vi "MasterAcquisitionFile_IOS_test.vi"() -> ()   [LabVIEW 2020]
uses:
  <vilib>/vision/driver/IMAQdx.llb/IMAQdx Acquisition Mode.ctl
  <vilib>/vision/driver/IMAQdx.llb/IMAQdx Camera Control Mode.ctl
  <vilib>/userDefined/High Color/IMAQdx.ctl
  <vilib>/vision/driver/IMAQdx.llb/IMAQdx Buffer Number Mode.ctl
  <vilib>/DAQmx/read.llb/DAQmx Read (Analog 1D Wfm NChan NSamp).vi
  <vilib>/Waveform/DWDTOps.llb/DWDT Digital to Boolean Array.vi
  <vilib>/DAQmx/create/channels.llb/DAQmx Create Channel (CO-Pulse Generation-Frequency).vi
  <vilib>/DAQmx/configure/timing.llb/DAQmx Timing (Implicit).vi
  <vilib>/DAQmx/create/channels.llb/DAQmx Create Channel (AI-Voltage-Basic).vi
  <vilib>/DAQmx/configure/timing.llb/DAQmx Timing (Sample Clock).vi
  <vilib>/DAQmx/configure/trigger.llb/DAQmx Start Trigger (Digital Edge).vi
  <vilib>/DAQmx/miscellaneous.llb/DAQmx Fill In Error Info.vi
  <vilib>/vision/driver/NI_Vision_Acquisition_Software.lvlib
  <resource>/objmgr/imaqdx.rc
panel:
  out "Saving":bool=TRUE
  in  "stop":bool
  in  "Sol Stim Parameters":cluster{"Fs":dbl, "Samples":dbl}
  in  "LED Stim Parameters":cluster{"Fs":dbl, "Samples":dbl}
  in  "Sol Duty Cycle (%)":dbl=10.0
  in  "Sol Freq":dbl=1.0
  in  "Sol Dur (s)":dbl=1.0
  in  "LED Duty Cycle (%)":dbl=10.0
  in  "LED Freq":dbl=10.0
  in  "LED Dur (s)":dbl=2.0
  out "Stimulus Order":digitalwaveform[](graph)=[{"t0"=timestamp(0 s since 1904-01-01), "dt"=5e-05, "Y"={"transitions"=[], "data"=array18001000x1[18001000 elements]}}, {"t0"=timestamp(0 s since 1904-01-01), "dt"=5e-05, "Y"={"transitions"=[], "data"=array18001000x1[18001000 elements]}}, {"t0"=timestamp(0 s since 1904-01-01), "dt"=5e-05, "Y"={"transitions"=[], "data"=array18001000x1[18001000 elements]}}, {"t0"=timestamp(0 s since 1904-01-01), "dt"=5e-05, "Y"={"transitions"=[], "data"=array18001000x1[18001000 elements]}}]
  out "Solenoid Stim":digitalwaveform(graph)={"t0"=timestamp(0 s since 1904-01-01), "dt"=5e-05, "Y"={"transitions"=[], "data"=array20000x1[20000 elements]}}
  in  "Trial Offset (s)":dbl=15.0
  in  "Interstim (s)":dbl=30.0
  in  "Right Pad":dbl=1.0
  in  "Left Pad":dbl=1.0
  in  "Auditory":dbl=1.0
  in  "LED":dbl
  out "?":T1(plugin-control)
  out "?":T1(plugin-control)
  out "Whisk Cam":bool=TRUE
  out "Web Cam":bool=TRUE
  out "Analog":bool=TRUE
  out "Web Cam Fs":dbl(knob)=29.86263189329086 scale=0.0..200.0
  out "Whisk Cam Fs":dbl(knob)=150.0 scale=0.0..200.0
  out "Dev1 Samples":i32=336839
  in  "Dev1 Analog Channels":string[](array[string])=["Cortical_LH", "Force_Sensor", "LPadSol", "RPadSol", "AudSol", "Hippocampus", "EMG", "Cortical_RH", "OptoLED"]
  in  "Analog Acquisition":cluster{"Analog Fs":u16}={"Analog Fs"=20000} {"Analog Fs" format="%0.0f"}
  in  "Sampling Rates":T2={"CBV Cam Fs"=30, "Whisk Cam Fs"=150, "Web Cam Fs"=30, "Pupil Cam Fs"=30}
  out "Notes Size":i32=8
  out "Notes Reversed":string[](array[string])=["Experimenter", "Animal ID", "Hemisphere", "Solenoid PSI", "Isoflurane time", "Session ID", "Amplifier Gain", "LED power (mW)"]
  out "Notes Array":string[](array[string])=["LED power (mW)", "Amplifier Gain", "Session ID", "Isoflurane time", "Solenoid PSI", "Hemisphere", "Animal ID", "Experimenter"]
  in  "Notes:":T3={"Experimenter"="Kevin", "Animal ID"="T195", "Hemisphere"="Both", "Solenoid PSI"="10", "Isoflurane time"="1130", "Session ID"="Imaging Session Five", "Amplifier Gain"="10000", "LED power (mW)"="10"}
  in  "Target Path":path=path "D:/T195/Imaging Session 5 - 5 June 2021" caption="Final Save Location"
  out "Dropped":u32(slide) caption="Whisk Cam" scale=0.0..999.0
  out "Filename":string="210605_11_36_30"
  in  "Time (min)":dbl(knob)=15.0 min=0.5 max=20.0 step=0.5 scale=0.0..20.0 scale format="%#_2g"
  in  "Temp Path":path=path "D:/LabVIEW Streamed Data" caption="Temporary Path for Streamed Data"
  out "Last Whisk\nBuffer":u32=2524
  # "Dropped Frames"
  # "Stimuli"
  # "LPAD"
  # "RPAD"
  # "AUD"
  # "LED"
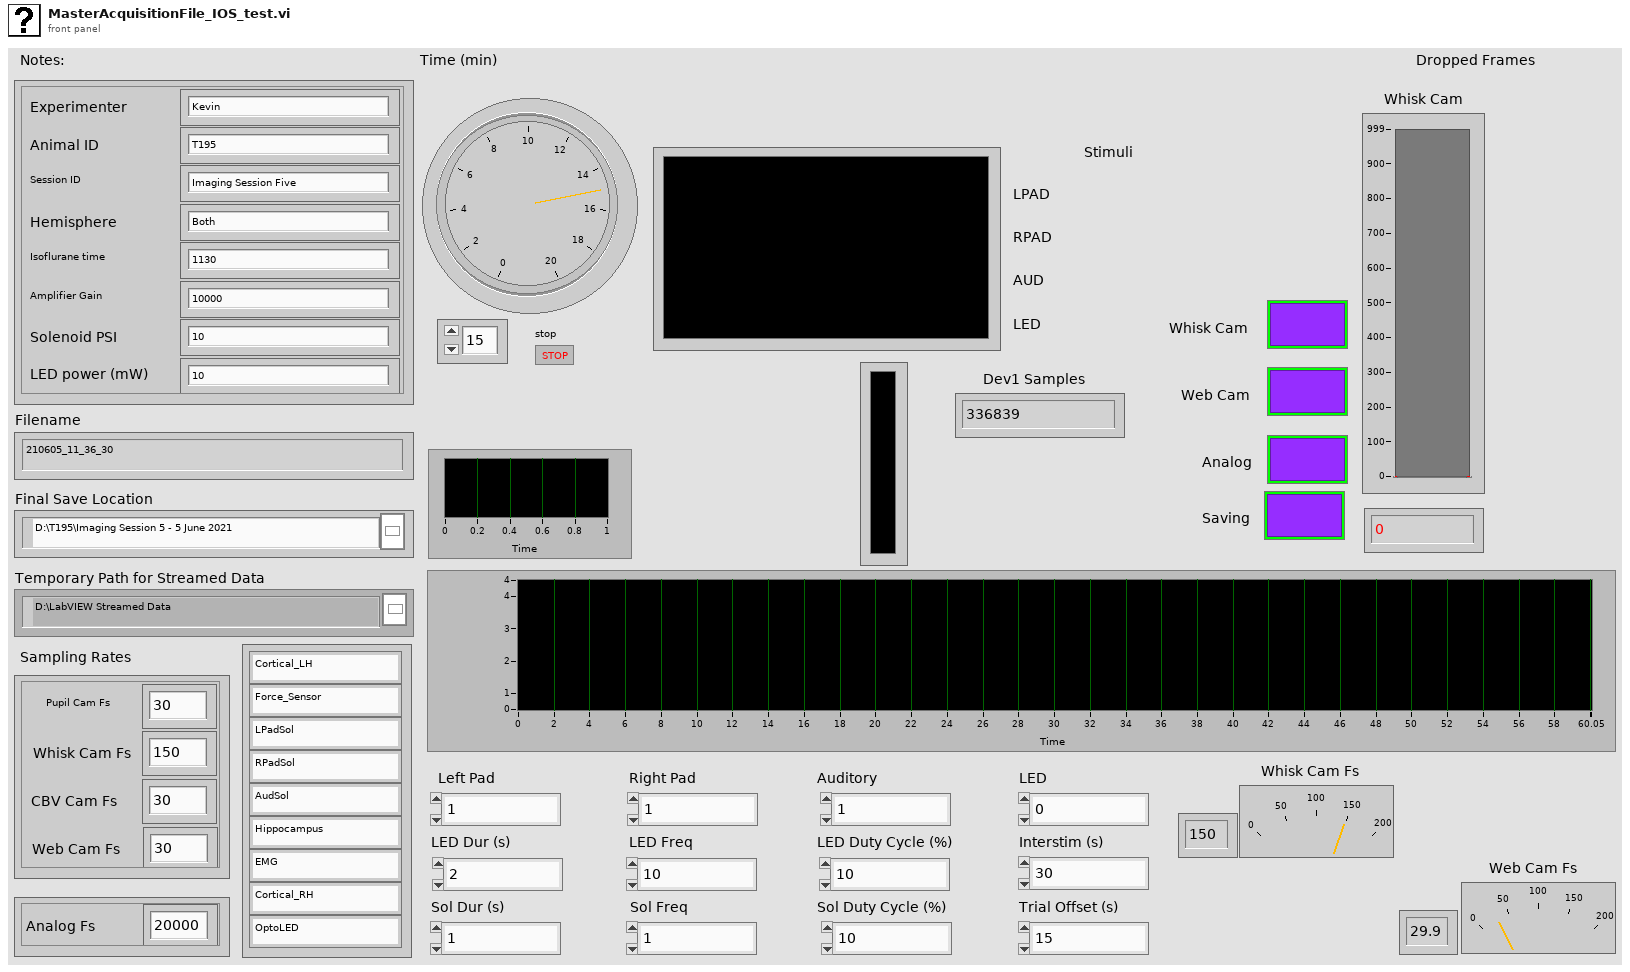
[diagram p1: front panel]
types:
  T1 = typedef "IMAQ Image.ctl" = refnum<image>
  T2 = cluster{"CBV Cam Fs":u16, "Whisk Cam Fs":u16, "Web Cam Fs":u16, "Pupil Cam Fs":u16}
  T3 = cluster{"Experimenter":string, "Animal ID":string, "Hemisphere":string, "Solenoid PSI":string, "Isoflurane time":string, "Session ID":string, "Amplifier Gain":string, "LED power (mW)":string}
  T4 = typedef "IMAQdx.ctl" = refnum<k21>
  T5 = enum16{"open", "open or create", "create or replace", "create", "open (read-only)"}
  T6 = typedef "Image Type" = u32
  T7 = typedef "NI_Vision_Acquisition_Software.lvlib/IMAQdx Camera Control Mode.ctl" = enum32{"Controller", "Listener"}
  T8 = enum16{"open", "replace", "create", "open or create", "replace or create", "replace or create with confirmation"}
  T9 = typedef "NI_Vision_Acquisition_Software.lvlib/IMAQdx Acquisition Mode.ctl" = enum32{"One Shot", "Continuous"}
  T10 = typedef "IMAQ AVI2 Refnum.ctl" = refnum<k20>
  T11 = enum16{"big-endian, network order", "native, host order", "little-endian"}
  T12 = typedef "NI_Vision_Acquisition_Software.lvlib/IMAQdx Buffer Number Mode.ctl" = enum32{"Next", "Last", "Buffer Number", "Every", "Last New"}
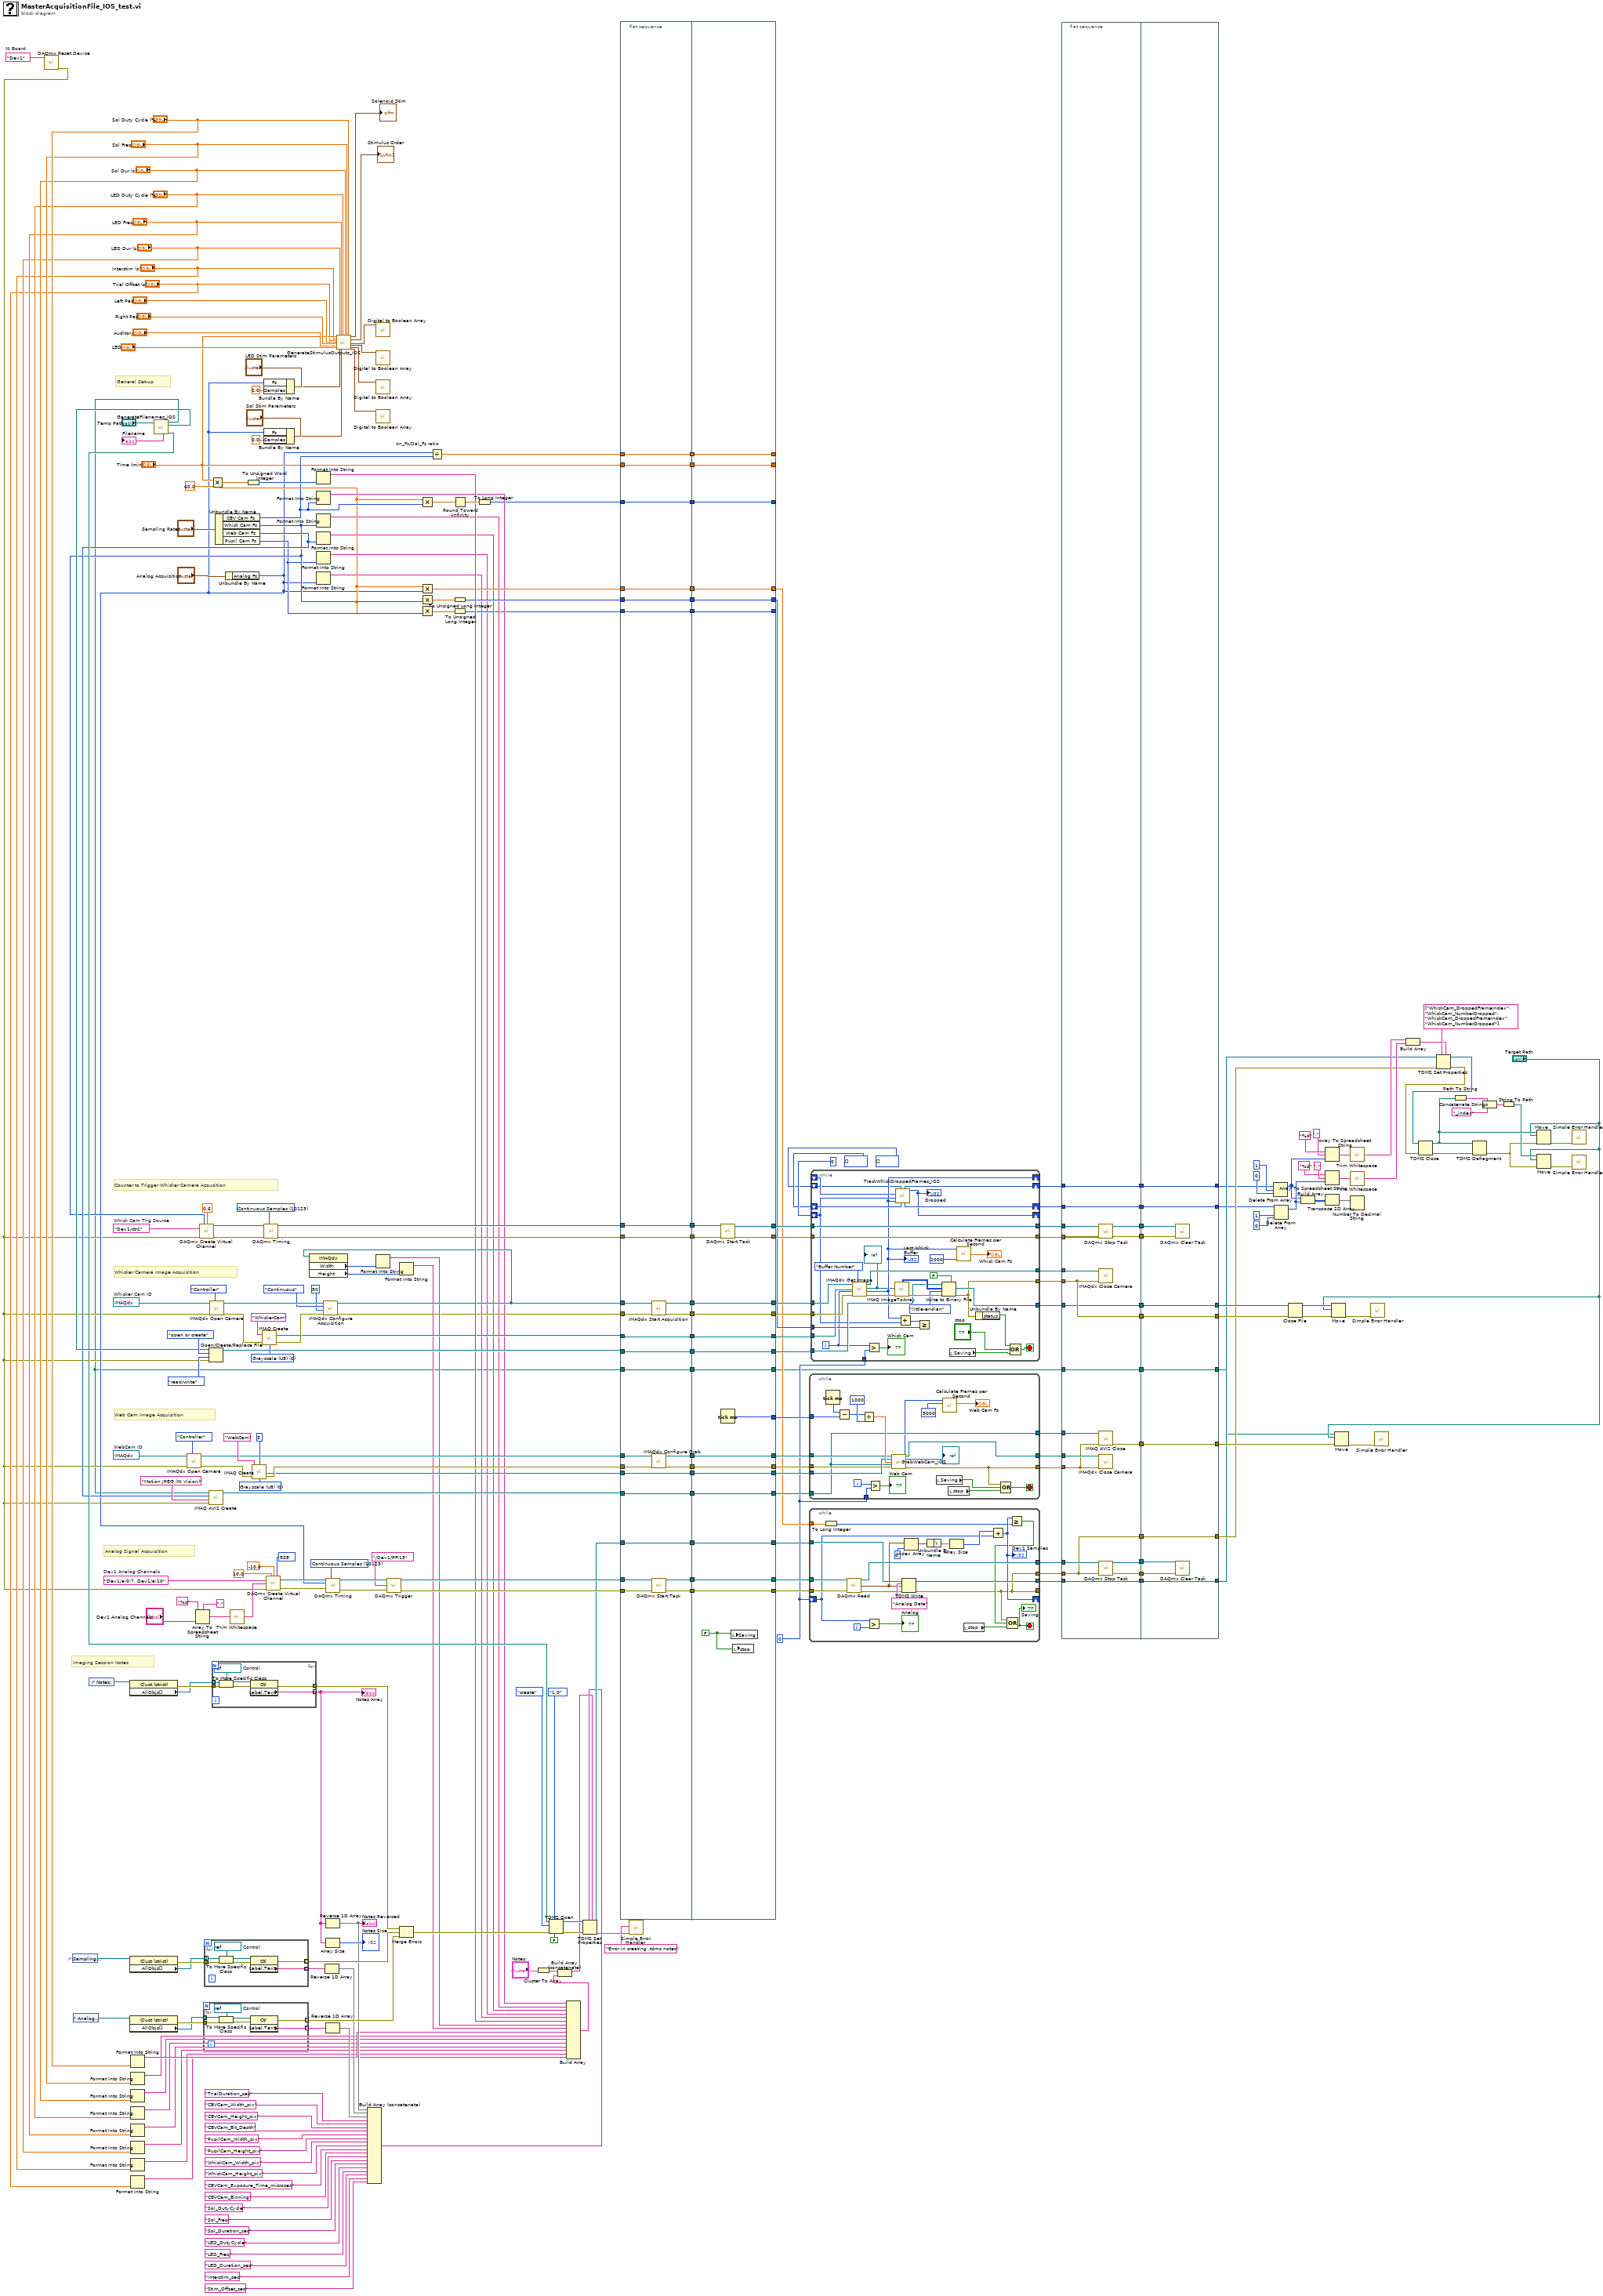
[diagram p0: block diagram]
diagram:
  w155 = tag "Dev1/ai0:7, Dev1/ai10"  # Dev1 Analog Channels
  w158 = T4 "cam0"  # WebCam ID
  w141 = T4 "cam1"  # Whisker Cam ID
  w268 = tag "Dev1/ctr1"  # Whisk Cam Trig Source
  w84 = 0
  w223 = 10123 items=["Finite Samples"=10178, "Continuous Samples"=10123, "Hardware Timed Single Point"=12522] ("sample mode")
  w226 = 10083 items=["default"=-1, "RSE"=10083, "NRSE"=10078, "Differential"=10106, "Pseudodifferential"=12529] ("input terminal configuration")
  w256 = T6 0 items=["Grayscale (U8)", "Grayscale (I16)", "Grayscale (SGL)", "Complex (CSG)", "RGB (U32)", "HSL (U32)", "RGB (U64)", "Grayscale (U16)"] ("Image Type")
  w263 = tag "Dev1"  # NI Board
  w264 = 10123 items=["Finite Samples"=10178, "Continuous Samples"=10123, "Hardware Timed Single Point"=12522] ("sample mode")
  w271 = T6 0 items=["Grayscale (U8)", "Grayscale (I16)", "Grayscale (SGL)", "Complex (CSG)", "RGB (U32)", "HSL (U32)", "RGB (U64)", "Grayscale (U16)"] ("Image Type")
  # "General Set-up"
  # "Whisker Camera Image Acquisition"
  # "Imaging Session Notes"
  # "Counter to Trigger Whisker Camera Acqusition"
  # "Web Cam Image Acquisition"
  # "Analog Signal Acquisition"
  n1 = call <vilib>:"DAQmx Reset Device.vi"("device in"=w263) -> ("error out"=w37:errorcluster)  [unwired: 14 in]
  n2 = control-ref of="Sampling Rates"() -> (w164:refnum<vi>)
  n3 = control-ref of="Analog Acquisition"() -> (w163:refnum<vi>)
  n4 = control-ref of="Notes:"() -> (w185:refnum<vi>)
  n5 = property class="Clust (strict)"(reference=w185) -> (error out=w188:errorcluster, "AllObjs[]"=w120:refnum<vi>[])  [unwired: 1 in, 1 out]
  n6 = property class="Clust (strict)"(reference=w164) -> (error out=w183:errorcluster, "AllObjs[]"=w121:refnum<vi>[])  [unwired: 1 in, 1 out]
  n7 = property class="Clust (strict)"(reference=w163) -> (error out=w162:errorcluster, "AllObjs[]"=w119:refnum<vi>[])  [unwired: 1 in, 1 out]
  n8 = Format Into String("Sol Duty Cycle (%)") -> (resulting string=w61:string)  [unwired: 3 in, 1 out]
  n9 = Format Into String("Sol Freq") -> (resulting string=w60:string)  [unwired: 3 in, 1 out]
  n10 = Format Into String("Sol Dur (s)") -> (resulting string=w59:string)  [unwired: 3 in, 1 out]
  n11 = Format Into String("LED Duty Cycle (%)") -> (resulting string=w58:string)  [unwired: 3 in, 1 out]
  n12 = Format Into String("LED Freq") -> (resulting string=w57:string)  [unwired: 3 in, 1 out]
  n13 = Format Into String("LED Dur (s)") -> (resulting string=w56:string)  [unwired: 3 in, 1 out]
  n14 = Format Into String("Interstim (s)") -> (resulting string=w55:string)  [unwired: 3 in, 1 out]
  n15 = Format Into String("Trial Offset (s)") -> (resulting string=w54:string)  [unwired: 3 in, 1 out]
  n16 = call "GenerateFilenames_IOS.vi"("path"="Temp Path") -> ("TDMS Path"=w180:path, "Basler Path"=w259:path, "WebCam Path"=w1:path, "Analog file name"=→"Filename":string)  [unwired: 3 in, 4 out]
  n17 = call <vilib>:"IMAQdx Open Camera.vi"("Camera Control Mode"=IMAQdx_Camera_Control_Mode."Controller", "error in"=w37, "Session In"=w158) -> ("error out"=w252:errorcluster, "Session Out"=w250:T4)  [unwired: 7 in]
  n18 = Array To Spreadsheet String(delimiter (Tab)=",", array="Dev1 Analog Channels", 3:"%s" ("format string")) -> (spreadsheet string=w152:string)
  n19 = for {
    tunnel: [w283] -> w160 mode=indexing
    tunnel: w162 -> [w282]
    tunnel: [w280] -> w161 mode=indexing
    tunnel: w119 -> [w279] mode=indexing
    w284 = refnum<vi> refnum  # Control
    n20 = To More Specific Class(target class=w284, reference=w279, error in=w282) -> (specific class reference=w285:refnum<vi>, error out=w281:errorcluster)
    n21 = property class="Ctl"(reference=w285, error in=w281) -> (error out=w280:errorcluster, "Label.Text"=w283:string)  [unwired: 1 out]
  }
  n22 = for {
    tunnel: [w290] -> w184 mode=indexing
    tunnel: w183 -> [w289]
    tunnel: [w287] -> w170 mode=indexing
    tunnel: w121 -> [w286] mode=indexing
    w291 = refnum<vi> refnum  # Control
    n23 = To More Specific Class(target class=w291, reference=w286, error in=w289) -> (specific class reference=w292:refnum<vi>, error out=w288:errorcluster)
    n24 = property class="Ctl"(reference=w292, error in=w288) -> (error out=w287:errorcluster, "Label.Text"=w290:string)  [unwired: 1 out]
  }
  n25 = Open/Create/Replace File(file path (use dialog)=w259, error in=w37, operation (0:open)=T8."open or create", access (0:read/write)=enum16{"read/write", "read-only", "write-only"}."read/write") -> (refnum out=w229:refnum<file>)  [unwired: 2 in, 2 out]
  n26 = call <vilib>:"IMAQdx Open Camera.vi"("Camera Control Mode"=IMAQdx_Camera_Control_Mode."Controller", "error in"=w37, "Session In"=w141) -> ("error out"=w274:errorcluster, "Session Out"=w277:T4)  [unwired: 7 in]
  n27 = Multiply(x="Time (min)", y=60.0) -> (x*y=w71:dbl)
  n28 = for {
    tunnel: [w297] -> w187 mode=indexing
    tunnel: w188 -> [w296]
    tunnel: [w294] -> w171 mode=indexing
    tunnel: w120 -> [w293] mode=indexing
    w298 = refnum<vi> refnum  # Control
    n29 = To More Specific Class(target class=w298, reference=w293, error in=w296) -> (specific class reference=w299:refnum<vi>, error out=w295:errorcluster)
    n30 = property class="Ctl"(reference=w299, error in=w295) -> (error out=w294:errorcluster, "Label.Text"=w297:string)  [unwired: 1 out]
  }
  "Notes Array" <- w187
  n31 = Unbundle By Name("Sampling Rates") -> ("CBV Cam Fs"=w72:u16, "Whisk Cam Fs"=w106:u16, "Web Cam Fs"=w157:u16, "Pupil Cam Fs"=w100:u16)
  n32 = call-poly <vilib>:"DAQmx Create Virtual Channel.vi"("frequency"=w106, "duty cycle"=0.6, "counter"=w268, "error in"=w37) -> ("task out"=w266:refnum<k21>, "error out"=w265:errorcluster)  [unwired: 10 in]
  n33 = call "IMAQ AVI2 Create"("error in (no error)"=w37, "Codec"="Motion JPEG (NI Vision)", "Frames Per Second"=w157, "AVI Path"=w1) -> ("AVI Refnum"=w242:T10)  [unwired: 6 in, 1 out]
  n34 = Unbundle By Name("Analog Acquisition") -> ("Analog Fs"=w45:u16)
  n35 = call <vilib>:"Trim Whitespace.vi"("string"=w152) -> ("trimmed string"=w151:string)  [unwired: 1 in]
  n36 = To Unsigned Word Integer(number=w71) -> (unsigned 16bit integer=w147:u16)
  n37 = call "IMAQ Create"("Border Size"=3, "Image Name"="WebCam", "Image Type"=w256, "error in (no error)"=w252) -> ("New Image"=w249:T1, "error out"=w251:errorcluster)  [unwired: 1 in]
  n38 = call "IMAQ Create"("Image Name"="WhiskerCam", "Image Type"=w271, "error in (no error)"=w274) -> ("New Image"=w139:T1, "error out"=w272:errorcluster)  [unwired: 2 in]
  n39 = Bundle By Name(cluster="LED Stim Parameters", "Fs"=w45, "Samples"=0.0) -> (w77:cluster{"Fs":dbl, "Samples":dbl})
  n40 = Bundle By Name(cluster="Sol Stim Parameters", "Fs"=w45, "Samples"=0.0) -> (w78:cluster{"Fs":dbl, "Samples":dbl})
  n41 = call-poly <vilib>:"DAQmx Timing.vi"("task/channels in"=w266, "sample mode"=w264, "error in"=w265) -> ("task out"=w213:refnum<k21>, "error out"=w211:errorcluster)  [unwired: 11 in]
  n42 = call-poly <vilib>:"DAQmx Create Virtual Channel.vi"("maximum value"=10.0, "minimum value"=-10.0, "input terminal configuration"=w226, "physical channels"=w155, "name to assign"=w151, "error in"=w37) -> ("task out"=w225:refnum<k21>, "error out"=w224:errorcluster)  [unwired: 8 in]
  n43 = Format Into String(w147) -> (resulting string=w149:string)  [unwired: 3 in, 1 out]
  n44 = Format Into String(w72) -> (resulting string=w104:string)  [unwired: 3 in, 1 out]
  n45 = Format Into String(w106) -> (resulting string=w103:string)  [unwired: 3 in, 1 out]
  n46 = Format Into String(w157) -> (resulting string=w102:string)  [unwired: 3 in, 1 out]
  n47 = Format Into String(w100) -> (resulting string=w90:string)  [unwired: 3 in, 1 out]
  n48 = Format Into String(w45) -> (resulting string=w89:string)  [unwired: 3 in, 1 out]
  n49 = call <vilib>:"IMAQdx Configure Acquisition.vi"("error in"=w272, "Number of Buffers"=u32 50, "Continuous?"=IMAQdx_Acquisition_Mode."Continuous", "Session In"=w277) -> ("error out"=w95:errorcluster, "Session Out"=w140:T4)  [unwired: 6 in]
  n50 = property class="IMAQdx"(reference=w140) -> ("Width"=w146:u32, "Height"=w145:u32)  [unwired: 1 in, 2 out]
  n51 = Reverse 1D Array(array=w184) -> (reversed array=w174:string[])
  n52 = Reverse 1D Array(array=w187) -> (reversed array=w118:string[])
  "Notes Reversed" <- w118
  n53 = Array Size(array=w187) -> (size(s)=→"Notes Size":i32)
  n54 = Reverse 1D Array(array=w160) -> (reversed array=w159:string[])
  n55 = call-poly <vilib>:"DAQmx Timing.vi"("task/channels in"=w225, "sample mode"=w223, "rate"=w45, "error in"=w224) -> ("task out"=w117:refnum<k21>, "error out"=w222:errorcluster)  [unwired: 10 in]
  n56 = call "GenerateStimulusOutputs_IOS.vi"("Trial duration (min)"="Time (min)", "Rest duration(s)"="Interstim (s)", "trial offset (s)"="Trial Offset (s)", "Left Pad"="Left Pad", "Right Pad"="Right Pad", "Auditory"="Auditory", "LED"="LED", "LED Stim Duration (s)"="LED Dur (s)", "LED Stim Parameters"=w77, "LED Frequency"="LED Freq", "Sol Stim Parameters"=w78, "LED duty cycle (%)"="LED Duty Cycle (%)", "Sol Stim Duration (s)"="Sol Dur (s)", "Sol Frequency"="Sol Freq", "Sol Duty Cycle (%)"="Sol Duty Cycle (%)") -> ("Solenoid Stim Waveforms"=→"Solenoid Stim":digitalwaveform, "Stimulus Digital Outputs"=→"Stimulus Order":digitalwaveform[], "Left Pad Out"=w44:digitalwaveform, "Auditory Out"=w43:digitalwaveform, "Right Pad Out"=w42:digitalwaveform, "LED Out"=w41:digitalwaveform)  [unwired: 7 in]
  n57 = Build Array (concatenate)(w118, w174, w159, "TrialDuration_sec", "CBVCam_Width_pix", "CBVCam_Height_pix", "CBVCam_Bit_Depth", "PupilCam_Width_pix", "PupilCam_Height_pix", "WhiskCam_Width_pix", "WhiskCam_Height_pix", "CBVCam_Exposure_Time_microsec" ("element"), "CBVCam_Binning" ("element"), "Sol_DutyCycle", "Sol_Freq", "Sol_Duration_sec", "LED_DutyCycle", "LED_Freq", "LED_Duration_sec", "Interstim_sec", "Stim_Offset_sec") -> (w115:string[])
  n58 = Format Into String(w146) -> (resulting string=w107:string)  [unwired: 3 in, 1 out]
  n59 = call-poly <vilib>:"Digital to Boolean Array.vi"("digital waveform"=w44) -> ()  [unwired: 9 in, 2 out]
  n60 = call-poly <vilib>:"Digital to Boolean Array.vi"("digital waveform"=w43) -> ()  [unwired: 9 in, 2 out]
  n61 = call-poly <vilib>:"Digital to Boolean Array.vi"("digital waveform"=w42) -> ()  [unwired: 9 in, 2 out]
  n62 = call-poly <vilib>:"Digital to Boolean Array.vi"("digital waveform"=w41) -> ()  [unwired: 9 in, 2 out]
  n63 = call-poly <vilib>:"DAQmx Trigger.vi"("task/channels in"=w117, "source"=tag "/Dev1/PFI13", "error in"=w222) -> ("task out"=w221:refnum<k21>, "error out"=w220:errorcluster)  [unwired: 11 in]
  n64 = Format Into String(w145) -> (resulting string=w108:string)  [unwired: 3 in, 1 out]
  n65 = Merge Errors(w171, w170, w161) -> (w169:errorcluster)
  n66 = Multiply(x=w71, y=w72) -> (x*y=w261:dbl)
  n67 = Multiply(x=w71, y=w45) -> (x*y=w130:dbl)
  n68 = Multiply(x=w106, y=w71) -> (x*y=w116:dbl)
  n69 = Multiply(x=w100, y=w71) -> (x*y=w105:dbl)
  n70 = Divide "An_Fs/Dal_Fs ratio"(x=w45, y=w72) -> (x/y=w39:dbl)
  n71 = To Unsigned Long Integer(number=w116) -> (unsigned 32bit integer=w128:u32)
  n72 = To Unsigned Long Integer(number=w105) -> (unsigned 32bit integer=w101:u32)
  n73 = Round Toward -Infinity(1:w261) -> (0:w260:dbl)
  n74 = To Long Integer(number=w260) -> (32bit integer=w96:i32)
  n75 = Cluster To Array(cluster="Notes:") -> (array=w181:string[])
  n76 = TDMS Open(6:FALSE ("disable buffering? (T)"), 7:enum16{"1.0", "2.0"}."1.0" ("file format version (2.0)"), 8:w169, 10:T5."create" ("operation (0:open)"), 11:w180) -> (0:w175:errorcluster, 3:w176:refnum<k34>)  [unwired: 2 in]
  n77 = Build Array(w104, w103, w102, w90, w89, w149, w107, w108, w61, w60, w59, w58, w57, w56, w55, w54) -> (w156:string[])
  n78 = Build Array (concatenate)(w181, w156) -> (w173:string[])
  n79 = TDMS Set Properties(5:w173, 7:w115, 8:w175, 11:w176) -> (0:w168:errorcluster, 3:w172:refnum<k34>)  [unwired: 2 in, 2 out]
  n80 = flat-sequence {
    tunnel: w251 -> [w325]
    tunnel: w250 -> [w324]
    tunnel: w249 -> [w323]
    tunnel: [w323] -> w248
    tunnel: [w322] -> w246
    tunnel: [w321] -> w244
    tunnel: w242 -> [w320]
    tunnel: [w320] -> w241
    tunnel: w140 -> [w319]
    tunnel: w95 -> [w318]
    tunnel: [w317] -> w236
    tunnel: [w316] -> w234
    tunnel: [w315] -> w232
    tunnel: w139 -> [w315]
    tunnel: [w314] -> w230
    tunnel: w229 -> [w314]
    tunnel: w96 -> [w313]
    tunnel: [w313] -> w228
    tunnel: "Time (min)" -> [w312]
    tunnel: [w312] -> w227
    tunnel: w221 -> [w311]
    tunnel: w220 -> [w310]
    tunnel: [w309] -> w219
    tunnel: [w308] -> w218
    tunnel: [w307] -> w214
    tunnel: w172 -> [w307]
    tunnel: w213 -> [w306]
    tunnel: [w306] -> w212
    tunnel: w211 -> [w305]
    tunnel: [w305] -> w210
    tunnel: w130 -> [w304]
    tunnel: [w304] -> w129
    tunnel: w128 -> [w303]
    tunnel: [w303] -> w127
    tunnel: w101 -> [w302]
    tunnel: [w302] -> w99
    tunnel: w39 -> [w301]
    tunnel: [w301] -> w38
    tunnel: w1 -> [w300]
    tunnel: [w300] -> w2
    tunnel: [w349] -> w253
    tunnel: w248 -> [w348]
    tunnel: [w348] -> w247
    tunnel: w246 -> [w347]
    tunnel: [w347] -> w245
    tunnel: w244 -> [w346]
    tunnel: [w346] -> w243
    tunnel: w241 -> [w345]
    tunnel: [w345] -> w240
    tunnel: [w335] -> w239
    tunnel: [w334] -> w238
    tunnel: [w344] -> w237
    tunnel: w236 -> [w344]
    tunnel: [w343] -> w235
    tunnel: w234 -> [w343]
    tunnel: [w342] -> w233
    tunnel: w232 -> [w342]
    tunnel: [w341] -> w231
    tunnel: w230 -> [w341]
    tunnel: w228 -> [w340]
    tunnel: [w340] -> _
    tunnel: [w339] -> _
    tunnel: w227 -> [w339]
    tunnel: [w338] -> w216
    tunnel: w219 -> [w338]
    tunnel: [w337] -> w217
    tunnel: w218 -> [w337]
    tunnel: [w336] -> w87
    tunnel: w214 -> [w336]
    tunnel: w212 -> [w333]
    tunnel: w210 -> [w332]
    tunnel: w129 -> [w331]
    tunnel: [w331] -> w88
    tunnel: w127 -> [w330]
    tunnel: [w330] -> w98
    tunnel: [w329] -> _
    tunnel: w99 -> [w329]
    tunnel: w38 -> [w328]
    tunnel: [w328] -> _
    tunnel: [w327] -> w4
    tunnel: w2 -> [w327]
    frame #0 {
      n81 = call <vilib>:"IMAQdx Start Acquisition.vi"("error in"=w318, "Session In"=w319) -> ("error out"=w316:errorcluster, "Session Out"=w317:T4)  [unwired: 8 in]
      n82 = call <vilib>:"IMAQdx Configure Grab.vi"("error in"=w325, "Session In"=w324) -> ("error out"=w321:errorcluster, "Session Out"=w322:T4)  [unwired: 8 in]
      n83 = call <vilib>:"DAQmx Start Task.vi"("task/channels in"=w311, "error in"=w310) -> ("task out"=w309:refnum<k21>, "error out"=w308:errorcluster)  [unwired: 12 in]
    }
    frame #1 {
      w326 = FALSE
      n84 = call <vilib>:"DAQmx Start Task.vi"("task/channels in"=w333, "error in"=w332) -> ("task out"=w335:refnum<k21>, "error out"=w334:errorcluster)  [unwired: 12 in]
      n85 = Tick Count (ms)() -> (millisecond timer value=w349:u32)
      n86 = local write "Saving"(w326) -> ()
      n87 = local write "stop"(w326) -> ()
    }
  }
  n88 = call <vilib>:"Simple Error Handler.vi"("error source (\" \")"="Error in creating .tdms notes" ("error source (\" \")"), "error in (no error)"=w168) -> ()  [unwired: 3 in, 5 out]
  n89 = while {
    tunnel: w217 -> [w371]
    tunnel: w216 -> [w370]
    tunnel: w87 -> [w369]
    tunnel: [w368] -> w13
    tunnel: [w358] -> _
    tunnel: [w367] -> w36
    shift-right: [w361] -> _
    shift-left: w84 -> [w353]
    tunnel: [w358] -> w35
    tunnel: w88 -> [w356]
    i -> [w354]
    stop <- w351 stop-if-true
    n90 = To Long Integer(number=w356) -> (32bit integer=w357:i32)
    n91 = call-poly <vilib>:"DAQmx Read.vi"("task/channels in"=w370, "error in"=w371) -> ("task out"=w367:refnum<k21>, "data"=w352:waveform(dbl)[], "error out"=w360:errorcluster)  [unwired: 11 in]
    n92 = Greater?(x=w353, y=w354) -> (0:→"Analog":bool)
    n93 = TDMS Write(0:w369, 5:"Analog Data" ("group name in (Untitled)"), 9:w352, 11:w360) -> (4:w368:refnum<k34>, 15:w358:errorcluster)  [unwired: 2 in, 2 out]
    n94 = Index Array(array=w352, index=0) -> (element=w364:waveform(dbl))
    n95 = Unbundle By Name(w364) -> ("Y"=w363:dbl[])
    n96 = Array Size(array=w363) -> (size(s)=w362:i32)
    n97 = local read "stop"() -> (w350:bool)
    n98 = Add(x=w362, y=w353) -> (x+y=w361:i32)
    "Dev1 Samples" <- w361
    n99 = Greater Or Equal?(x=w361, y=w357) -> (x >= y?=w359:bool)
    n100 = Compound Arithmetic op=OR(w358, w359, w350) -> (w351:bool)
    "Saving" <- w351
  }
  n101 = while {
    tunnel: w253 -> [w388]
    tunnel: w247 -> [w386]
    tunnel: w245 -> [w385]
    tunnel: w243 -> [w384]
    tunnel: w240 -> [w382]
    tunnel: [w383] -> w27
    tunnel: [w375] -> w28
    tunnel: [w382] -> w26
    tunnel: w84 -> [w377]
    i -> [w378]
    stop <- w376 stop-if-true
    n102 = Tick Count (ms)() -> (millisecond timer value=w390:u32)
    n103 = Subtract(x=w390, y=w388) -> (x-y=w391:u32)
    n104 = Divide(x=w391, y=u32 1000) -> (x/y=w387:dbl)
    n105 = Greater?(x=w378, y=w377) -> (0:→"Web Cam":bool)
    n106 = call "GrabWebCam_IOS.vi"("Session In"=w385, "Image In"=w386, "Trial Time"=w387, "AVI Refnum"=w382, "error in"=w384) -> ("Session Out"=w383:T4, "WebCam Img Out"=→"?":T1, "Buffer Number Out"=w381:u32, "error out"=w375:errorcluster)  [unwired: 7 in]
    n107 = local read "Saving"() -> (w373:bool)
    n108 = call <vilib>:"Calculate Frames per Second.vi"("Update Interval (ms)"=u32 5000, "Buffer Number"=w381) -> ("Processed Frames/s"=→"Web Cam Fs":dbl)  [unwired: 7 in, 2 out]
    n109 = local read "stop"() -> (w372:bool)
    n110 = Compound Arithmetic op=OR(w375, w373, w372) -> (w376:bool)
  }
  n111 = while {
    tunnel: w239 -> [w419]
    tunnel: [w420] -> w31
    tunnel: w238 -> [w420]
    tunnel: [w419] -> w32
    tunnel: [w412] -> w22
    tunnel: [w413] -> w23
    tunnel: [w418] -> w18
    tunnel: w237 -> [w417]
    tunnel: w235 -> [w416]
    tunnel: w233 -> [w415]
    tunnel: w231 -> [w414]
    shift-right: [w403] -> _
    shift-left: _ -> [w401]
    shift-right: [w398] -> _
    shift-left: u32 0 ("New Lost") -> [w402]
    shift-right: [w399] -> w8
    shift-left: u32[] [] ("NewBuffNum") -> [w400]
    shift-right: [w405] -> w11
    shift-left: u32[] [] ("NewNumLost") -> [w404]
    tunnel: w98 -> [w410]
    tunnel: w84 -> [w406]
    i -> [w395]
    stop <- w409 stop-if-true
    n112 = call <vilib>:"IMAQdx Get Image.vi"("Buffer Number Mode (Next)"=IMAQdx_Buffer_Number_Mode."Buffer Number", "error in"=w416, "Buffer Number In"=w395, "Image In"=w415, "Session In"=w417) -> ("error out"=w426:errorcluster, "Buffer Number Out"=w403:u32, "Image Out"=w397:T1, "Session Out"=w412:T4)  [unwired: 3 in]
    "Last Whisk\nBuffer" <- w403
    "?" <- w397
    n113 = Greater?(x=w395, y=w406) -> (0:→"Whisk Cam":bool)
    n114 = call "IMAQ ImageToArray"("error in (no error)"=w426, "Image"=w397) -> ("error out"=w425:errorcluster, "Image Pixels (U8)"=w424:u8[][])  [unwired: 2 in, 3 out]
    n115 = call "TrackWhiskDroppedFrames_IOS.vi"("NumLost"=w404, "BuffNum"=w400, "Curr Buffer"=w403, "Prev Lost"=w402, "Prev Buffer"=w401) -> ("New Lost"=w398:u32, "NewNumLost"=w405:u32[], "NewBuffNum"=w399:u32[])  [unwired: 4 in]
    "Dropped" <- w398
    n116 = Add(x=w403, y=w402) -> (x+y=w411:u32)
    n117 = Greater Or Equal?(x=w411, y=w410) -> ()  [unwired: 1 out]
    n118 = Write to Binary File(file (use dialog)=w414, data=w424, error in=w425, 5:FALSE ("prepend array or string size? (T)"), 9:T11."little-endian" ("byte order (0:big-endian, network order)")) -> (refnum out=w418:refnum<file>, error out=w413:errorcluster)  [unwired: 1 in, 1 out]
    n119 = local read "Saving"() -> (w393:bool)
    n120 = call <vilib>:"Calculate Frames per Second.vi"("Update Interval (ms)"=u32 2000, "Buffer Number"=w403) -> ("Processed Frames/s"=→"Whisk Cam Fs":dbl)  [unwired: 7 in, 2 out]
    n121 = Unbundle By Name(w413) -> ("status"=w396:bool)
    n122 = Compound Arithmetic op=OR(w396, "stop", w393) -> (w409:bool)
  }
  n123 = flat-sequence {
    tunnel: w36 -> [w446]
    tunnel: w35 -> [w432]
    tunnel: [w445] -> w34
    tunnel: [w444] -> w33
    tunnel: w32 -> [w443]
    tunnel: w31 -> [w442]
    tunnel: [w441] -> _
    tunnel: [w440] -> _
    tunnel: [w441] -> w30
    tunnel: [w440] -> w29
    tunnel: w28 -> [w438]
    tunnel: w27 -> [w439]
    tunnel: w26 -> [w437]
    tunnel: [w436] -> w25
    tunnel: w23 -> [w434]
    tunnel: w22 -> [w435]
    tunnel: [w434] -> w20
    tunnel: [w433] -> w19
    tunnel: w18 -> [w433]
    tunnel: [w432] -> w16
    tunnel: w13 -> [w431]
    tunnel: [w431] -> w14
    tunnel: w11 -> [w430]
    tunnel: [w430] -> w10
    tunnel: w8 -> [w429]
    tunnel: [w429] -> w7
    tunnel: w4 -> [w428]
    tunnel: [w428] -> w3
    tunnel: w34 -> [w458]
    tunnel: w33 -> [w457]
    tunnel: w30 -> [w456]
    tunnel: w29 -> [w455]
    tunnel: w25 -> [w454]
    tunnel: [w454] -> w24
    tunnel: [w453] -> w21
    tunnel: w20 -> [w453]
    tunnel: w19 -> [w452]
    tunnel: [w452] -> w17
    tunnel: w16 -> [w451]
    tunnel: [w451] -> w15
    tunnel: w14 -> [w450]
    tunnel: [w450] -> w12
    tunnel: w10 -> [w449]
    tunnel: [w449] -> w9
    tunnel: [w448] -> w6
    tunnel: w7 -> [w448]
    tunnel: [w447] -> w5
    tunnel: w3 -> [w447]
    frame #0 {
      n124 = call <vilib>:"DAQmx Stop Task.vi"("task/channels in"=w443, "error in"=w442) -> ("task out"=w441:refnum<k21>, "error out"=w440:errorcluster)  [unwired: 12 in]
      n125 = call <vilib>:"IMAQdx Close Camera.vi"("error in"=w434, "Session In"=w435) -> ()  [unwired: 9 in, 1 out]
      n126 = call "IMAQ AVI2 Close"("error in (no error)"=w438, "AVI Refnum"=w437) -> ("error out"=w436:errorcluster)  [unwired: 9 in]
      n127 = call <vilib>:"IMAQdx Close Camera.vi"("error in"=w438, "Session In"=w439) -> ()  [unwired: 9 in, 1 out]
      n128 = call <vilib>:"DAQmx Stop Task.vi"("task/channels in"=w446, "error in"=w432) -> ("task out"=w445:refnum<k21>, "error out"=w444:errorcluster)  [unwired: 12 in]
    }
    frame #1 {
      n129 = call <vilib>:"DAQmx Clear Task.vi"("task in"=w456, "error in"=w455) -> ()  [unwired: 13 in, 1 out]
      n130 = call <vilib>:"DAQmx Clear Task.vi"("task in"=w458, "error in"=w457) -> ()  [unwired: 13 in, 1 out]
    }
  }
  n131 = Delete From Array(array=w6, length=1, index=0) -> (array with subset deleted=w123:u32[])  [unwired: 1 out]
  n132 = Delete From Array(array=w9, length=1, index=0) -> (array with subset deleted=w124:u32[])  [unwired: 1 out]
  n133 = Close File(refnum=w17, error in=w21) -> (path=w201:path, error out=w200:errorcluster)
  n134 = Build Array(w123, w124) -> (w126:u32[][])
  n135 = Array To Spreadsheet String(delimiter (Tab)=",", array=w124, 3:"%d" ("format string")) -> (spreadsheet string=w131:string)
  n136 = Transpose 2D Array(2D array=w126) -> (transposed array=w125:u32[][])
  n137 = Array To Spreadsheet String(delimiter (Tab)=",", array=w123, 3:"%d" ("format string")) -> (spreadsheet string=w132:string)
  n138 = Move(source path=w201, error in=w200, 10:"Target Path") -> (error out=w198:errorcluster)  [unwired: 2 in, 2 out]
  n139 = Move(source path=w5, error in=w24, 10:"Target Path") -> (error out=w197:errorcluster)  [unwired: 2 in, 2 out]
  n140 = call <vilib>:"Trim Whitespace.vi"("string"=w132) -> ("trimmed string"=w93:string)  [unwired: 1 in]
  n141 = call <vilib>:"Trim Whitespace.vi"("string"=w131) -> ("trimmed string"=w92:string)  [unwired: 1 in]
  n142 = Number To Decimal String(number=w125) -> ()  [unwired: 1 in, 1 out]
  n143 = call <vilib>:"Simple Error Handler.vi"("error in (no error)"=w198) -> ()  [unwired: 1 in, 8 out]
  n144 = call <vilib>:"Simple Error Handler.vi"("error in (no error)"=w197) -> ()  [unwired: 1 in, 8 out]
  n145 = Build Array(w93, w92) -> (w91:string[])
  n146 = TDMS Set Properties(5:w91, 7:string[] ["WhiskCam_DroppedFrameIndex", "WhiskCam_NumberDropped", "WhiskCam_DroppedFrameIndex", "WhiskCam_NumberDropped"] ("channel name(s) in (Untitled)"), 8:w15, 11:w12) -> (0:w138:errorcluster, 3:w137:refnum<k34>)  [unwired: 2 in, 2 out]
  n147 = TDMS Close(8:w138, 11:w137) -> (0:w202:errorcluster, 3:w194:path)
  n148 = Path To String(path=w194) -> (string=w196:string)
  n149 = TDMS Defragment(4:w202, 7:w194) -> (0:w191:errorcluster)
  n150 = Concatenate Strings(w196, "_index" ("string")) -> (w193:string)
  n151 = String To Path(string=w193) -> (path=w192:path)
  n152 = Move(source path=w194, error in=w191, 10:"Target Path") -> (error out=w199:errorcluster)  [unwired: 2 in, 2 out]
  n153 = Move(source path=w192, error in=w191, 10:"Target Path") -> (error out=w97:errorcluster)  [unwired: 2 in, 2 out]
  n154 = call <vilib>:"Simple Error Handler.vi"("error in (no error)"=w199) -> ()  [unwired: 1 in, 8 out]
  n155 = call <vilib>:"Simple Error Handler.vi"("error in (no error)"=w97) -> ()  [unwired: 1 in, 8 out]
